vi "StateMachine.vi"() -> ()   [LabVIEW 2020]
uses:
  <vilib>/ErrorRing/Error Ring.xnode
panel:
  in  "stop":bool
  in  "ALRM":dbl(slide) scale=0.0..100.0
  out "String":string
  in  "Nombre del Archivo":string
  in  "Formato":string(combo)
  in  "Direccion":path
  out "Array 2":bool[](array[boolean])
  out "Array":dbl[](array[slide]) scale=0.0..100.0
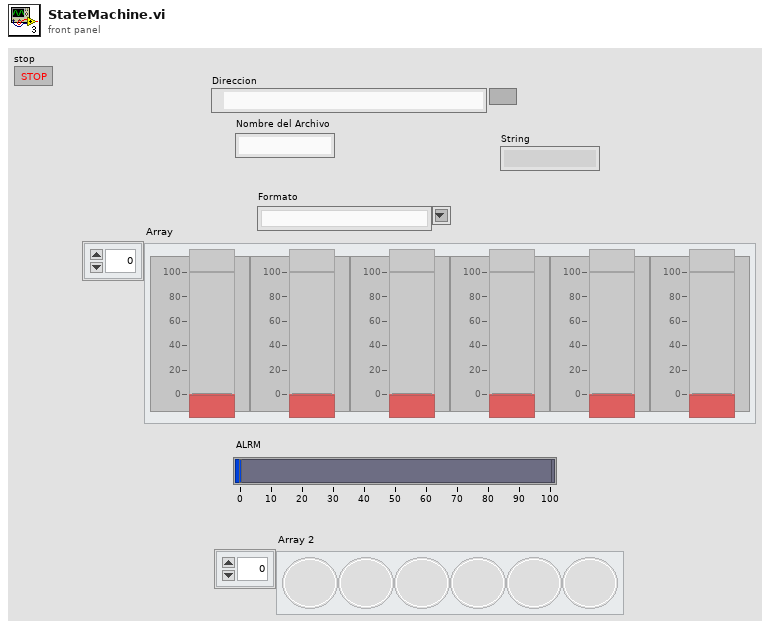
[diagram p1: front panel]
types:
  T1 = cluster{"Data_Analisis":cluster{"Direccion":path, "NombreArchivo":string, "refnum out":refnum<file>, "Formato ":string}, "N_Valores":cluster{"N_elementos":i32, "L_MAX":dbl, "L_MIN":dbl}, "Hardware":cluster{"Data_value":dbl[]}, "Warning":cluster{"Alarma":bool[]}}
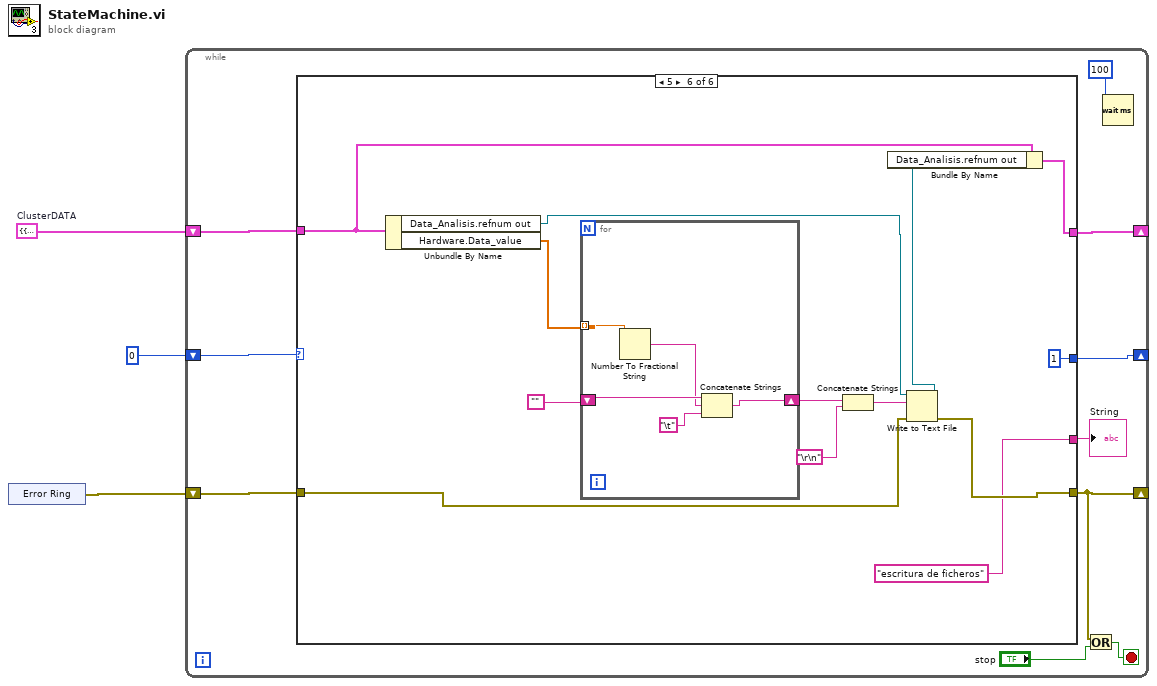
[diagram p0: block diagram]
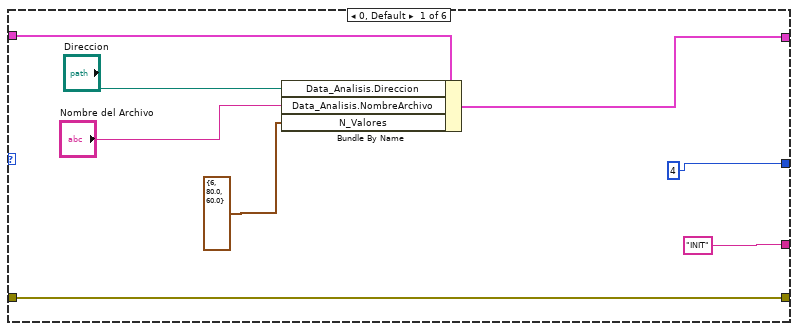
[diagram p2: hidden frame]
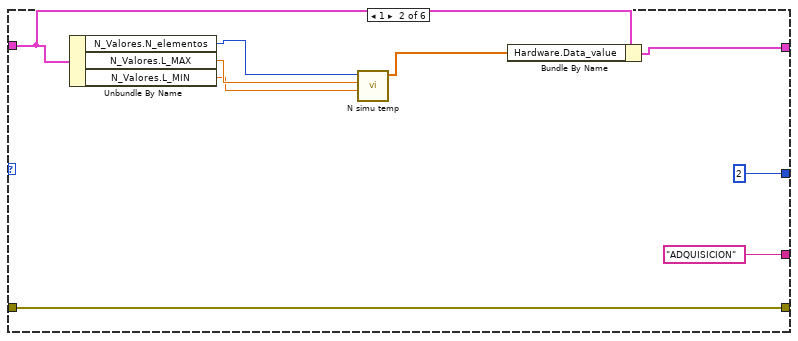
[diagram p3: hidden frame]
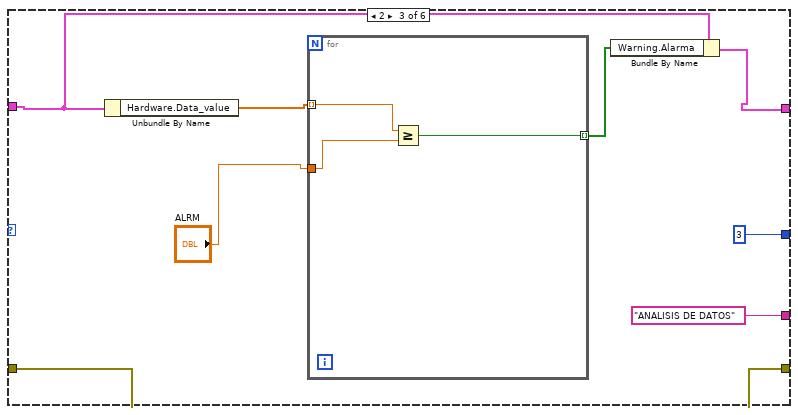
[diagram p4: hidden frame]
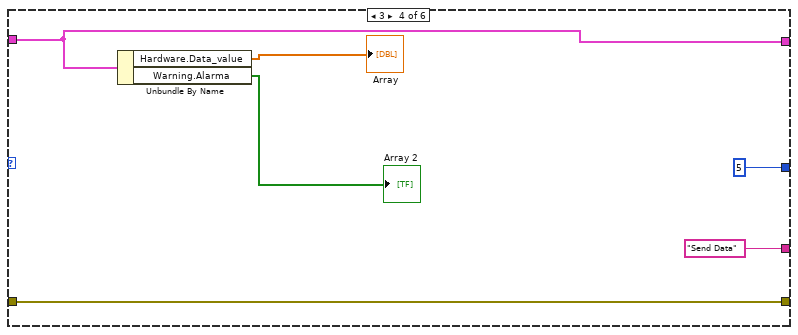
[diagram p5: hidden frame]
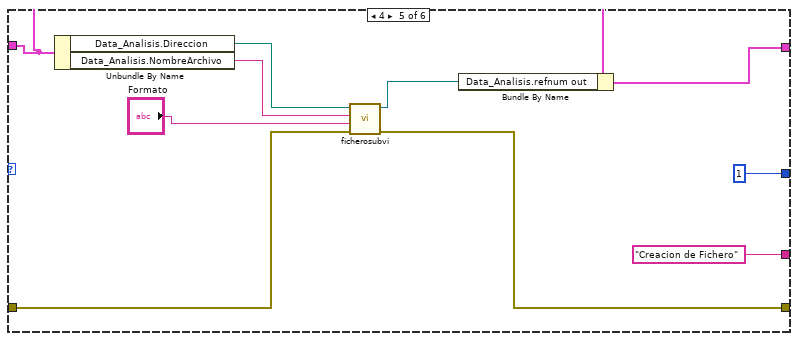
[diagram p6: hidden frame]
diagram:
  w2 = T1 {"Data_Analisis"={"Direccion"=path "", "NombreArchivo"="", "refnum out"=refnum, "Formato "=""}, "N_Valores"={"N_elementos"=0, "L_MAX"=0.0, "L_MIN"=0.0}, "Hardware"={"Data_value"=[]}, "Warning"={"Alarma"=[FALSE]}}  # ClusterDATA
  n1 = xnode "Error Ring"() -> ("error out"=w1:errorcluster)
  n2 = while {
    shift-right: [w10] -> _
    shift-left: 0 -> [w13]
    shift-right: [w11] -> _
    shift-left: w2 -> [w12]
    shift-right: [w5] -> _
    shift-left: w1 -> [w8]
    stop <- w7 stop-if-true
    n3 = case shown="5" w13 {
      tunnel: w12 -> [w21 w27 w36 w45 w52 w62]
      tunnel: [w17 w25 w35 w45 w50 w60] -> w11
      tunnel: [4 2 3 5 1 1] -> w10
      tunnel: ["INIT" "ADQUISICION" "ANALISIS DE DATOS" "Send Data" "Creacion de Fichero" "escritura de ficheros"] -> w9
      tunnel: w8 -> [w14 w24 w33 w43 w54 w64]
      tunnel: [w14 w24 w33 w43 w53 w63] -> w5
      frame 0, Default {
        n4 = Bundle By Name(cluster=w21, "Data_Analisis.Direccion"="Direccion", "Data_Analisis.NombreArchivo"="Nombre del Archivo", "N_Valores"=cluster{i32, dbl, dbl} {6, 80.0, 60.0}) -> (w17:T1)
      }
      frame 1 {
        n5 = Unbundle By Name(w27) -> ("N_Valores.N_elementos"=w30:i32, "N_Valores.L_MAX"=w29:dbl, "N_Valores.L_MIN"=w28:dbl)
        n6 = call "N simu temp.vi"("Limite Minimo"=w28, "Limite Maximo"=w29, "Numeric"=w30) -> ("Array"=w26:dbl[])  [unwired: 8 in]
        n7 = Bundle By Name(cluster=w27, "Hardware.Data_value"=w26) -> (w25:T1)
      }
      frame 2 {
        n8 = Unbundle By Name(w36) -> ("Hardware.Data_value"=w38:dbl[])
        n9 = for {
          tunnel: w38 -> [w41] mode=indexing
          tunnel: "ALRM" -> [w40]
          tunnel: [w39] -> w34 mode=indexing
          n10 = Greater Or Equal?(x=w41, y=w40) -> (x >= y?=w39:bool)
        }
        n11 = Bundle By Name(cluster=w36, "Warning.Alarma"=w34) -> (w35:T1)
      }
      frame 3 {
        n12 = Unbundle By Name(w45) -> ("Hardware.Data_value"=→"Array":dbl[], "Warning.Alarma"=→"Array 2":bool[])
      }
      frame 4 {
        n13 = Unbundle By Name(w52) -> ("Data_Analisis.Direccion"=w57:path, "Data_Analisis.NombreArchivo"=w56:string)
        n14 = call "ficherosubvi.vi"("error in (no error)"=w54, "Formato"="Formato", "Nombre del Archivo"=w56, "Direccion"=w57) -> ("error out"=w53:errorcluster, "Byte Stream File out"=w51:refnum<file>)  [unwired: 6 in]
        n15 = Bundle By Name(cluster=w52, "Data_Analisis.refnum out"=w51) -> (w50:T1)
      }
      frame 5 {
        n16 = Unbundle By Name(w62) -> ("Data_Analisis.refnum out"=w65:refnum<file>, "Hardware.Data_value"=w70:dbl[])
        n17 = for {
          tunnel: w70 -> [w75] mode=indexing
          shift-right: [w71] -> w68
          shift-left: "" -> [w74]
          n18 = Number To Fractional String(number=w75) -> (F-format string=w73:string)  [unwired: 3 in]
          n19 = Concatenate Strings(w74, w73, "\t") -> (w71:string)
        }
        n20 = Concatenate Strings(w68, "\r\n") -> (w66:string)
        n21 = Write to Text File(file (use dialog)=w65, text=w66, error in=w64) -> (refnum out=w61:refnum<file>, error out=w63:errorcluster)  [unwired: 1 in, 1 out]
        n22 = Bundle By Name(cluster=w62, "Data_Analisis.refnum out"=w61) -> (w60:T1)
      }
    }
    "String" <- w9
    n23 = Or(x=w5, y="stop") -> (x .or. y?=w7:bool)
    n24 = Wait (ms)(milliseconds to wait=u32 100) -> ()  [unwired: 1 out]
  }
